vi "CAN-RefreshListbox.vi"(6 "Table":refnum<vi>, 8 "Values":sgl[](array[numeric]), 11 "FramesInfo":T1) -> (0 "IDs":sgl[](array[numeric]), 3 "FramesInfo":T1)   [LabVIEW 2016]
uses:
  Shared/Typedefs/System-CAN-FrameInfoArray.ctl
  Shared/Typedefs/System-CAN-FrameInfo.ctl
  <vilib>/addons/Software Calibration Management/xSCM/Controls/ID and Element.ctl
  <vilib>/Utility/miscctls.llb/LVRowAndColumnTypeDef.ctl
  <vilib>/addons/Software Calibration Management/xSCM/SCM-API.lvlib
  Shared/DSI-Shared.lvlib
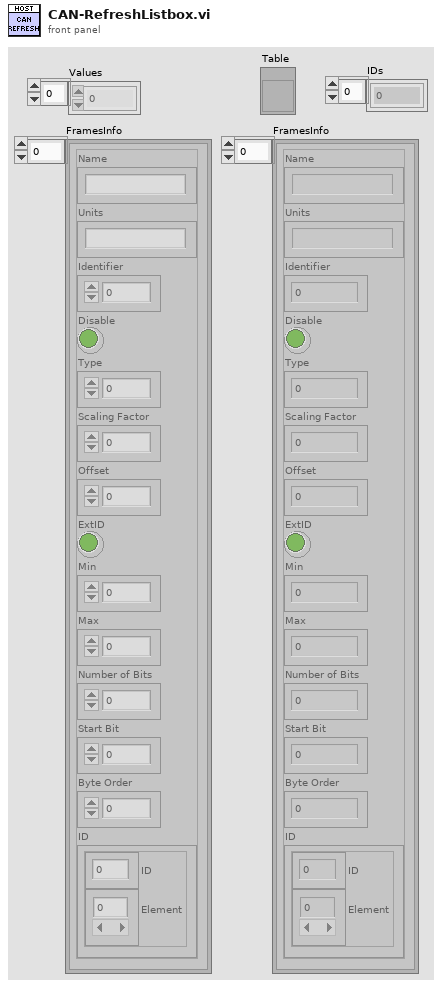
[diagram p1: front panel]
types:
  T1 = typedef "DSI-Shared.lvlib/System-CAN-FrameInfoArray.ctl" = T2[]
  T2 = typedef "DSI-Shared.lvlib/System-CAN-FrameInfo.ctl" = cluster{"Name":string, "Units":string, "Identifier":u32, "Disable":bool, "Type":u8, "Scaling Factor":sgl, "Offset":sgl, "ExtID":bool, "Min":sgl, "Max":sgl, "Number of Bits":u8, "Start Bit":u8, "Byte Order":u8, "ID":T3}
  T3 = typedef "SCM-API.lvlib/ID and Element.ctl" = cluster{"ID":u32, "Element":i32[]}
  T4 = typedef "LVRowAndColumnTypeDef.ctl" = cluster{"Row":i32, "Column":i32}
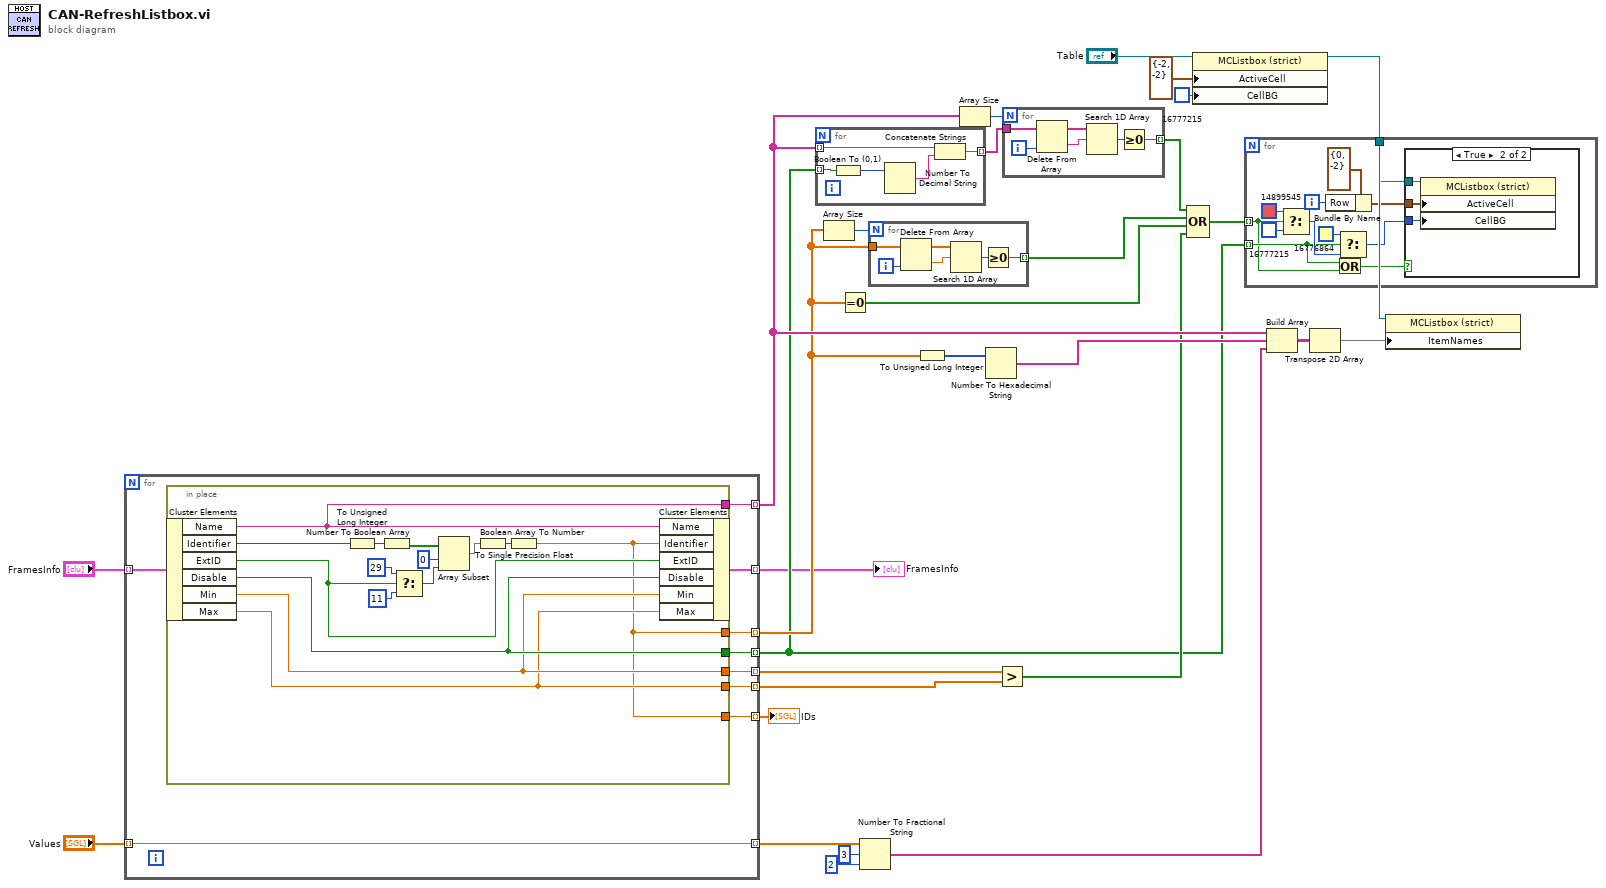
[diagram p0: block diagram]
diagram:
  n1 = for {
    tunnel: [w34] -> w8 mode=indexing
    tunnel: [w35] -> w9 mode=indexing
    tunnel: [w36] -> w5 mode=indexing
    tunnel: [w37] -> w17 mode=indexing
    tunnel: [w38] -> w13 mode=indexing
    tunnel: "FramesInfo" -> [w33] mode=indexing
    tunnel: [w32] -> w4 mode=indexing
    tunnel: [w31] -> w3 mode=indexing
    tunnel: "Values" -> [w30] mode=indexing
    tunnel: [w30] -> w1 mode=indexing
    n2 = in-place {
      in-place-border: [w39] -> w38
      in-place-border: [w44] -> w37
      in-place-border: [w42] -> w36
      in-place-border: [w41] -> w35
      in-place-border: [w40] -> w34
      in-place-border: [w39] -> w31
      n3 = in-place-cluster #1(w33) -> ("Name"=w44:string, "Identifier"=w45:u32, "ExtID"=w43:bool, "Disable"=w42:bool, "Min"=w41:sgl, "Max"=w40:sgl)
      n4 = To Unsigned Long Integer(number=w45) -> (unsigned 32bit integer=w53:u32)
      n5 = Number To Boolean Array(number=w53) -> (Boolean array=w52:bool[])
      n6 = Select(t=29 ("index"), s=w43, f=11 ("index")) -> (s? t:f=w50:i32)
      n7 = Array Subset(array=w52, index=0, length=w50) -> (w46:bool[])
      n8 = Boolean Array To Number(Boolean array=w46) -> (number=w47:u32)
      n9 = To Single Precision Float(number=w47) -> (single precision float=w39:sgl)
      n10 = in-place-cluster #1("Name"=w44, "Identifier"=w39, "ExtID"=w43, "Disable"=w42, "Min"=w41, "Max"=w40) -> (w32:T2)
    }
  }
  "FramesInfo" <- w4
  "IDs" <- w3
  n11 = for {
    tunnel: [w56] -> w18 mode=indexing
    tunnel: w17 -> [w57] mode=indexing
    tunnel: w5 -> [w55] mode=indexing
    n12 = Boolean To (0,1)(Boolean=w55) -> (0, 1=w54:i16)
    n13 = Number To Decimal String(number=w54) -> (decimal integer string=w58:string)  [unwired: 1 in]
    n14 = Concatenate Strings(w57, w58) -> (w56:string)
  }
  n15 = Array Size(array=w13) -> (size(s)=w27:i32)
  n16 = Equal To 0?(x=w13) -> (x = 0?=w16:bool[])
  n17 = Number To Fractional String(number=w1, width (-)=i16 3, precision (6)=i16 2) -> (F-format string=w12:string[])  [unwired: 1 in]
  n18 = for {
    N: w27 -> [_]
    tunnel: w13 -> [w63]
    tunnel: [w59] -> w25 mode=indexing
    i -> [w62]
    n19 = Delete From Array(array=w63, index=w62) -> (deleted portion=w60:sgl, array with subset deleted=w61:sgl[])  [unwired: 1 in]
    n20 = Search 1D Array(1D array=w61, element=w60) -> (index of element=w64:i32)  [unwired: 1 in]
    n21 = Greater Or Equal To 0?(x=w64) -> (x >= 0?=w59:bool)
  }
  n22 = To Unsigned Long Integer(number=w13) -> (unsigned 32bit integer=w14:u32[])
  n23 = Array Size(array=w17) -> (size(s)=w28:i32)
  n24 = Number To Hexadecimal String(2:w14) -> (0:w19:string[])  [unwired: 1 in]
  n25 = Greater?(x=w9, y=w8) -> (0:w7:bool[])
  n26 = for {
    N: w28 -> [_]
    tunnel: w18 -> [w65]
    tunnel: [w68] -> w26 mode=indexing
    i -> [w66]
    n27 = Delete From Array(array=w65, index=w66) -> (deleted portion=w69:string, array with subset deleted=w67:string[])  [unwired: 1 in]
    n28 = Search 1D Array(1D array=w67, element=w69) -> (index of element=w70:i32)  [unwired: 1 in]
    n29 = Greater Or Equal To 0?(x=w70) -> (x >= 0?=w68:bool)
  }
  n30 = Compound Arithmetic op=OR(w26, w25, w16, w7) -> (w24:bool[])
  n31 = property on="Property Node" class="MCListbox (strict)"(reference="Table", "ActiveCell"=T4 {"Row"=-2, "Column"=-2} ("Active Cell:Active Cell"), "CellBG"=u32 16777215 ("Color Box")) -> (reference out=w20:refnum<vi>)  [unwired: 1 in, 1 out]
  n32 = for {
    tunnel: w20 -> [w80]
    tunnel: w24 -> [w72] mode=indexing
    tunnel: w5 -> [w73] mode=indexing
    i -> [w77]
    n33 = Select(t=u32 14899545 ("Color Box"), s=w72, f=u32 16777215 ("Color Box")) -> (s? t:f=w76:u32)
    n34 = Bundle By Name(cluster=T4 {"Row"=0, "Column"=-2} ("Active Cell:Active Cell"), "Row"=w77) -> (w81:T4)
    n35 = Or(x=w73, y=w72) -> (x .or. y?=w71:bool)
    n36 = Select(t=u32 16776864 ("Color Box"), s=w73, f=w76) -> (s? t:f=w75:u32)
    n37 = case shown="True" w71 {
      tunnel: w81 -> [_ w85]
      tunnel: w80 -> [_ w84]
      tunnel: w75 -> [_ w83]
      frame False {
      }
      frame True {
        n38 = property on="Property Node" class="MCListbox (strict)"(reference=w84, "ActiveCell"=w85, "CellBG"=w83) -> ()  [unwired: 1 in, 2 out]
      }
    }
  }
  n39 = Build Array(w17, w19, w12) -> (w15:string[][])
  n40 = Transpose 2D Array(2D array=w15) -> (transposed array=w29:string[][])
  n41 = property on="Property Node" class="MCListbox (strict)"(reference=w20, "ItemNames"=w29) -> ()  [unwired: 1 in, 2 out]
